vi "WriterMyRio.vi"(2 "Leistung":dbl, 3 "Drehzahl":dbl, 4 "Arraysensor":bool[](array[boolean])=[FALSE, FALSE, FALSE, FALSE, FALSE, FALSE, FALSE, FALSE], 5 "IR Sensoren":dbl[](array[numeric])) -> (0 "Output":dbl[](array[numeric]))   [LabVIEW 2016]
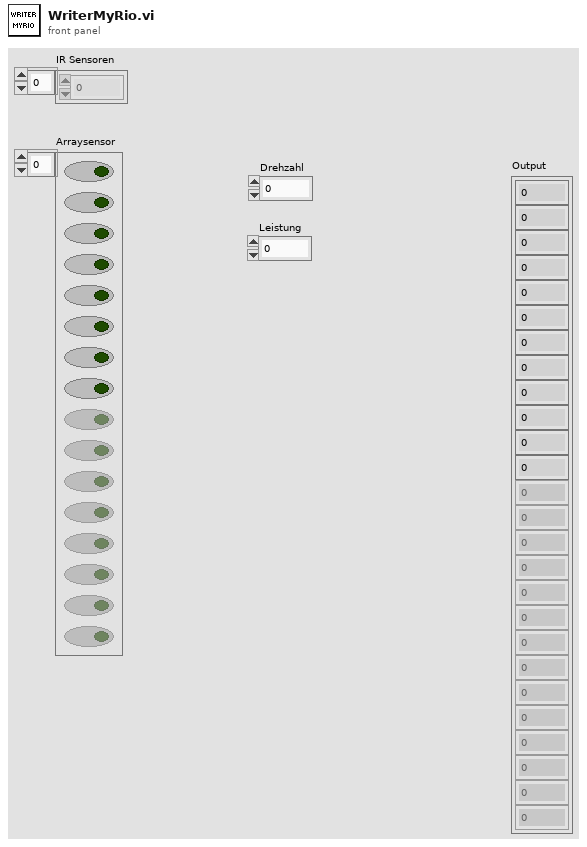
[diagram p1: front panel]
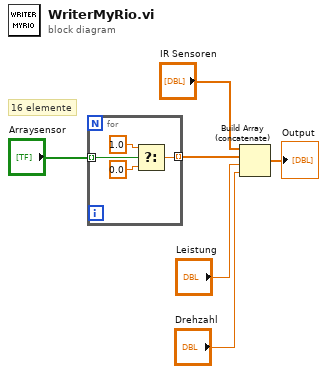
[diagram p0: block diagram]
diagram:
  # "16 elemente"
  n1 = for {
    tunnel: "Arraysensor" -> [w8] mode=indexing
    tunnel: [w7] -> w5 mode=indexing
    n2 = Select(t=1.0, s=w8, f=0.0) -> (s? t:f=w7:dbl)
  }
  n3 = Build Array (concatenate)("IR Sensoren", w5, "Leistung", "Drehzahl") -> (→"Output":dbl[])
